vi "习题3.4.vi"() -> ()   [LabVIEW 2018]
panel:
  out "长度":i32
  out "字符串 3":string
  out "字符串 2":string
  out "字符串":string
  out "连接的字符串":string
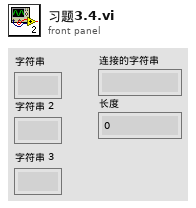
[diagram p1: front panel]
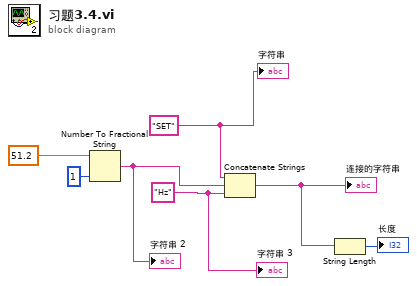
[diagram p0: block diagram]
diagram:
  w4 = "Hz" ("字符串")
  w3 = "SET" ("字符串")
  n1 = Number To Fractional String(number=51.2 ("数字"), precision (6)=i16 1 ("精度(6)")) -> (F-format string=w5:string)  [unwired: 2 in]
  "字符串 2" <- w5
  n2 = Concatenate Strings(w3, w5, w4) -> (w2:string)
  "连接的字符串" <- w2
  n3 = String Length(string=w2) -> (length=→"长度":i32)
  "字符串" <- w3
  "字符串 3" <- w4
